vi "BG-singleexp-correctSD.vi"(1 "def pixel upper":dbl, 4 "group":i32, 5 "def pixel lower":dbl, 6 "error in (no error)":errorcluster, 7 "exp selected":i32, 8 "Experiments groups":refnum<class "Experiments_group.lvclass">[](array[class]), 9 "Commentaires":refnum<vi>) -> (0 "error out":errorcluster, 2 "Experiments groups out":refnum<class "Experiments_group.lvclass">[](array[class]), 3 "Array":dbl[][](array[numeric]))   [LabVIEW 2015]
uses:
  Classes/Experiments_group.lvclass
  Classes/Experiment.lvclass
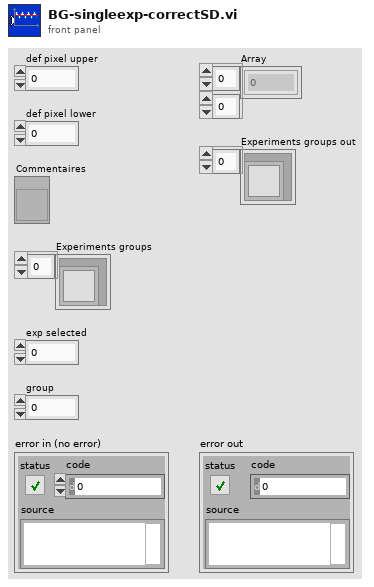
[diagram p1: front panel]
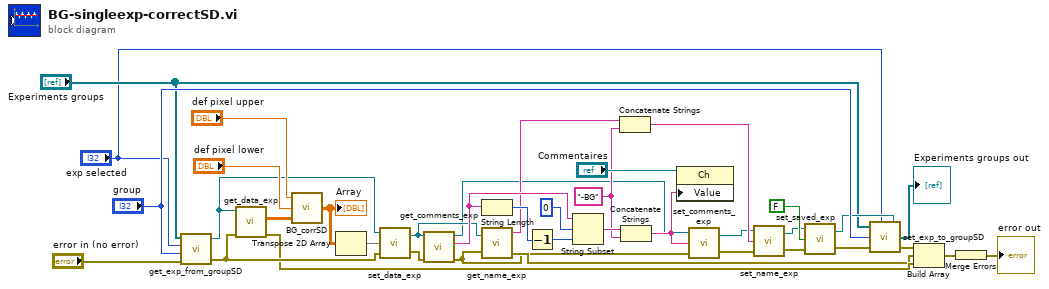
[diagram p0: block diagram]
diagram:
  w20 = "-BG" ("string")
  n1 = call "get_exp_from_groupSD.vi"("error in (no error)"="error in (no error)", "group"="group", "exp selected"="exp selected", "Experiments groups"="Experiments groups") -> ("error out"=w28:errorcluster, "Experiment out"=w25:refnum<class "Experiment.lvclass">)  [unwired: 1 out]
  n2 = call-dynamic "get_data_exp.vi"("error in (no error)"=w28, "Experiment.lvclass in"=w25) -> ("error out"=w27:errorcluster, "Data"=w26:dbl[][])  [unwired: 7 in, 1 out]
  n3 = call "BG_corrSD.vi"("Data"=w26, "lower pixel"="def pixel lower", "upper pixel"="def pixel upper") -> ("Array"=w24:dbl[][])
  "Array" <- w24
  n4 = Transpose 2D Array(2D array=w24) -> (transposed array=w23:dbl[][])
  n5 = call-dynamic "set_data_exp.vi"("error in (no error)"=w28, "Data"=w23, "Experiment.lvclass in"=w25) -> ("error out"=w3:errorcluster, "Experiment.lvclass out"=w13:refnum<class "Experiment.lvclass">)
  n6 = call-dynamic "get_comments_exp.vi"("error in (no error)"=w3, "Experiment.lvclass in"=w13) -> ("error out"=w14:errorcluster, "Comments"=w33:string, "Experiment.lvclass out"=w4:refnum<class "Experiment.lvclass">)  [unwired: 7 in]
  n7 = String Length(string=w33) -> (length=w35:i32)
  n8 = call-dynamic "get_name_exp.vi"("Experiment.lvclass in"=w13, "error in (no error)"=w14) -> ("Exp name"=w19:string, "error out"=w16:errorcluster)  [unwired: 1 out]
  n9 = Decrement(x=w35) -> (x-1=w36:i32)
  n10 = String Subset(string=w33, offset (0)=0, length (rest)=w36) -> (substring=w37:string)
  n11 = Concatenate Strings(w19, w20) -> (w21:string)
  n12 = Concatenate Strings(w37, w20) -> (w5:string)
  n13 = property on="Property Node" class="Ch"(reference="Commentaires", "Value"=w5) -> ()  [unwired: 1 in, 2 out]
  n14 = call-dynamic "set_comments_exp.vi"("error in (no error)"=w14, "Comments"=w5, "Experiment.lvclass in"=w4) -> ("error out"=w10:errorcluster, "Experiment.lvclass out"=w8:refnum<class "Experiment.lvclass">)
  n15 = call-dynamic "set_name_exp.vi"("error in (no error)"=w10, "Exp name"=w21, "Experiment.lvclass in"=w8) -> ("error out"=w12:errorcluster, "Experiment.lvclass out"=w11:refnum<class "Experiment.lvclass">)
  n16 = call-dynamic "set_saved_exp.vi"("error in (no error)"=w12, "Saved"=FALSE, "Experiment.lvclass in"=w11) -> ("error out"=w15:errorcluster, "Experiment.lvclass out"=w9:refnum<class "Experiment.lvclass">)
  n17 = call "set_exp_to_groupSD.vi"("Experiments groups"="Experiments groups", "exp selected"="exp selected", "group"="group", "error in (no error)"=w15, "Experiment in"=w9) -> ("Experiments groups out"=→"Experiments groups out":refnum<class "Experiments_group.lvclass">[], "error out"=w17:errorcluster)  [unwired: 1 in]
  n18 = Build Array(w17, w16, w27) -> (w38:errorcluster[])
  n19 = Merge Errors(w38) -> (→"error out":errorcluster)
